vi "rs3_2D Plane fit_sub2.vi"(6 "algorithm":T1 items=["SVD", "Givens", "Givens2", "Householder", "LU Decomposition", "Cholesky", "SVD for Rank Deficient H"], 7 "method":T2 items=["Least Square", "Least Absolute Residual", "Bisquare"], 9 "Pointcloud Z":dbl[][](array[numeric]), 10 "Pointcloud Y":dbl[][](array[numeric]), 11 "Pointcloud X":dbl[][](array[numeric])) -> (0 "Coefficients":dbl[](array[numeric])=[5.057324840764333, 0.002760084925691242, -0.016560509554140346], 1 "mean Z Value":dbl=5.04447078879859 format="%0.2f", 2 "rms error value":dbl=0.06652497327232935 format="%0.4f", 3 "rms %":dbl=1.3187701159862044 format="%0.4f", 4 "Deviation":dbl[](array[numeric])=[-0.060084925690023994, 0.037154989384283965, 0.03439490445859228, 0.05647558386411511, -0.14628450106157498, 0.05095541401273351, 0.07303609341825634, -0.029723991507434988, -0.01592356687898544], 5 "Best Fit":dbl[](array[numeric])=[5.060084925690024, 5.062845010615716, 5.065605095541407, 5.0435244161358845, 5.046284501061575, 5.049044585987266, 5.026963906581743, 5.029723991507435, 5.015923566878985])   [LabVIEW 2017, in "libRealSense3.lvlib"]
uses:
  <vilib>/Analysis/6fits.llb/Curve Fitting Criteria.ctl
  <vilib>/Analysis/6fits.llb/General Linear Fit Algorithm.ctl
  <vilib>/Analysis/5stat.llb/RMS (DBL).vi
  <vilib>/Analysis/baseanly.llb/Mean (DBL).vi
  <vilib>/Math Plots/3D Math Plots/3D Scatter/3D Scatter Datatype/Public/Plot Helper (Vector).vi
  libRealSense3.lvlib
  <vilib>/Math Plots/3D Math Plots/3D Scatter/3D Scatter Datatype/3D Scatter Datatype.lvclass
  <vilib>/Analysis/NI_AALPro.lvlib
  <vilib>/Analysis/NI_AALBase.lvlib
panel:
  out "AngleY":dbl=1.3187701159862044 format="%0.8f"
  out "AngleX":dbl=1.3187701159862044 format="%0.8f"
  # "INPUT DATA"
  # "PLANE FIT"
  # "Z= A +B*x+C*y"
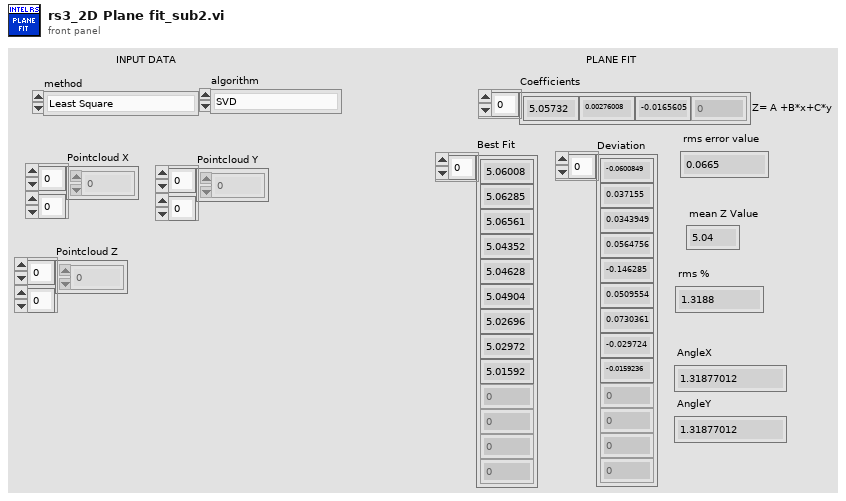
[diagram p1: front panel]
types:
  T1 = typedef "NI_AALPro.lvlib/General Linear Fit Algorithm.ctl" = u16
  T2 = typedef "NI_AALPro.lvlib/Curve Fitting Criteria.ctl" = u16
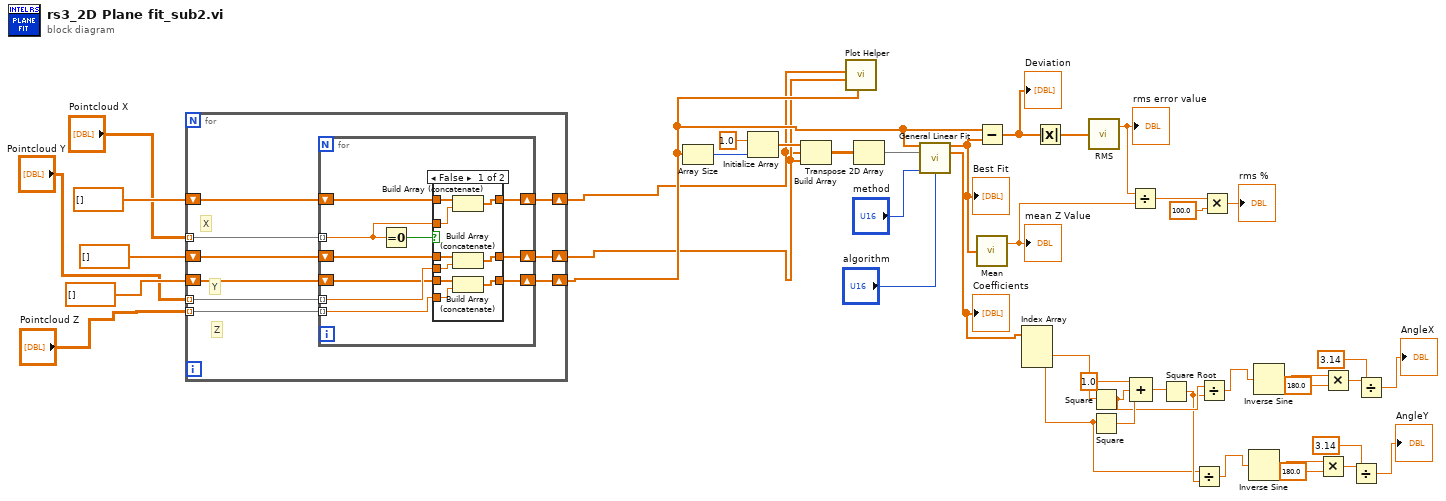
[diagram p0: block diagram]
diagram:
  n1 = for {
    tunnel: "Pointcloud X" -> [w53] mode=indexing
    tunnel: "Pointcloud Y" -> [w52] mode=indexing
    tunnel: "Pointcloud Z" -> [w51] mode=indexing
    shift-right: [w50] -> w21
    shift-left: dbl[] [] -> [w47]
    shift-right: [w48] -> w22
    shift-left: dbl[] [] -> [w46]
    shift-right: [w49] -> w23
    shift-left: dbl[] [] -> [w45]
    # "Z"
    # "Y"
    # "X"
    n2 = for {
      tunnel: w53 -> [w62] mode=indexing
      tunnel: w52 -> [w59] mode=indexing
      tunnel: w51 -> [w58] mode=indexing
      shift-right: [w61] -> w50
      shift-left: w47 -> [w60]
      shift-right: [w55] -> w48
      shift-left: w46 -> [w54]
      shift-right: [w56] -> w49
      shift-left: w45 -> [w57]
      n3 = Equal To 0?(x=w62) -> (x = 0?=w63:bool)
      n4 = case shown="False" w63 {
        tunnel: w62 -> [w72 _]
        tunnel: [w71 w75] -> w61
        tunnel: w60 -> [w70 w75]
        tunnel: w59 -> [w69 _]
        tunnel: w58 -> [w68 _]
        tunnel: w57 -> [w67 w73]
        tunnel: [w66 w73] -> w56
        tunnel: [w65 w74] -> w55
        tunnel: w54 -> [w64 w74]
        frame False {
          n5 = Build Array (concatenate)(w70, w72) -> (w71:dbl[])
          n6 = Build Array (concatenate)(w64, w69) -> (w65:dbl[])
          n7 = Build Array (concatenate)(w67, w68) -> (w66:dbl[])
        }
        frame True {
        }
      }
    }
  }
  n8 = Array Size(array=w23) -> (size(s)=w44:i32)
  n9 = Initialize Array(1.0 ("element"), w44) -> (w42:dbl[])
  n10 = Build Array(w42, w21, w22) -> (w30:dbl[][])
  n11 = call-poly <vilib>:"Plot Helper.vi"("z vector"=w23, "y vector"=w22, "x vector"=w21) -> ()  [unwired: 3 in, 6 out]
  n12 = Transpose 2D Array(2D array=w30) -> (transposed array=w41:dbl[][])
  n13 = call <vilib>:"General Linear Fit.vi"("Y"=w23, "H"=w41, "method"="method", "algorithm"="algorithm") -> ("Best Fit"=w36:dbl[], "Coefficients"=w20:dbl[])  [unwired: 6 in, 4 out]
  "Best Fit" <- w36
  "Coefficients" <- w20
  n14 = Subtract(x=w23, y=w36) -> (x-y=w38:dbl[])
  "Deviation" <- w38
  n15 = call-poly <vilib>:"Mean.vi"("X"=w36) -> ("mean"=w34:dbl)  [unwired: 1 out]
  "mean Z Value" <- w34
  n16 = Index Array(array=w20) -> (element #2=w19:dbl, element #3=w2:dbl)  [unwired: 3 in, 1 out]
  n17 = Absolute Value(x=w38) -> (abs(x)=w37:dbl[])
  n18 = call-poly <vilib>:"RMS.vi"("X"=w37) -> ("rms value"=w35:dbl)  [unwired: 1 out]
  "rms error value" <- w35
  n19 = Square(x=w19) -> (x^2=w10:dbl)
  n20 = Square(x=w2) -> (x^2=w17:dbl)
  n21 = Divide(x=w35, y=w34) -> (x/y=w33:dbl)
  n22 = Compound Arithmetic op=ADD(1.0 ("value"), w10, w17) -> (w18:dbl)
  n23 = Square Root(x=w18) -> (sqrt(x)=w3:dbl)
  n24 = Divide(x=w2, y=w3) -> (x/y=w4:dbl)
  n25 = Divide(x=w10, y=w3) -> (x/y=w16:dbl)
  n26 = Multiply(x=w33, y=100.0) -> (x*y=→"rms %":dbl)
  n27 = Inverse Sine(1:w4) -> (0:w5:dbl)
  n28 = Inverse Sine(1:w16) -> (0:w15:dbl)
  n29 = Multiply(x=w5, y=180.0) -> (x*y=w7:dbl)
  n30 = Multiply(x=w15, y=180.0) -> (x*y=w13:dbl)
  n31 = Divide(x=w7, y=3.14) -> (x/y=→"AngleY":dbl)
  n32 = Divide(x=w13, y=3.14) -> (x/y=→"AngleX":dbl)
